vi "Segment Waveform Array.vi"(8 "error in (no error)":errorcluster caption="错误输入（无错误）", 10 "segment time":dbl=5.0 caption="分割时刻" format="%#_13g", 11 "original wavefrom array":waveform(dbl)[](array[waveform]) caption="原波形数组") -> (0 "error out":errorcluster caption="错误输出", 2 "waveform array part 0":waveform(dbl)[](array[waveform]) caption="波形数组前段", 3 "waveform array part 1":waveform(dbl)[](array[waveform]) caption="波形数组后段")   [LabVIEW 2015]
uses:
  <vilib>/Waveform/WDTOps.llb/WDT Waveform Duration DBL.vi
  <vilib>/Waveform/WDTOps.llb/WDT Get Waveform Subset DBL.vi
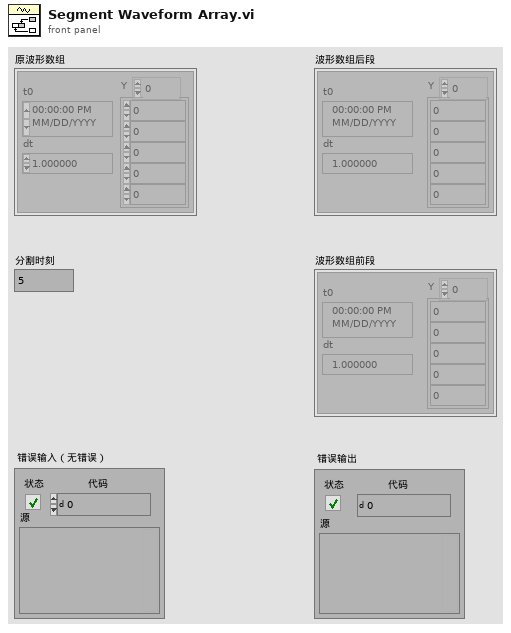
[diagram p1: front panel]
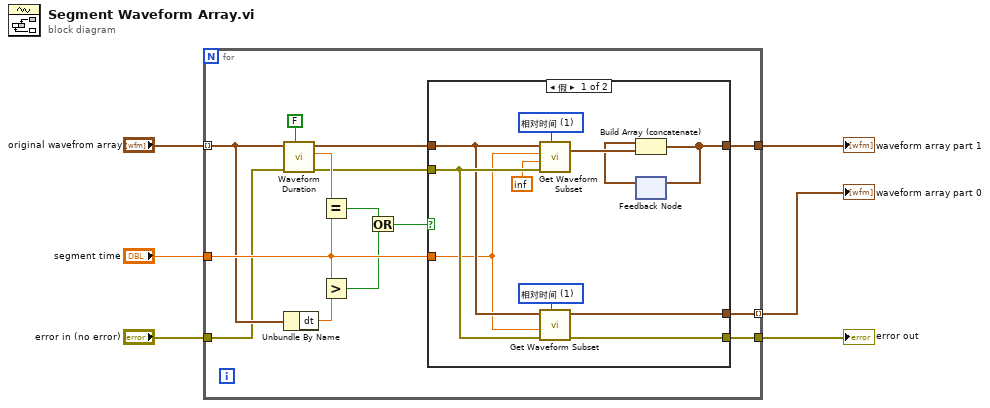
[diagram p0: block diagram]
diagram:
  n1 = for {
    tunnel: [w20] -> w4 mode=indexing
    tunnel: "original wavefrom array" -> [w10] mode=indexing
    tunnel: "error in (no error)" -> [w9]
    tunnel: [w19] -> w6
    tunnel: [w7] -> w1
    tunnel: "segment time" -> [w15]
    n2 = call-poly <vilib>:"Waveform Duration.vi"("open interval? (T)"=FALSE, "error in (no error)"=w9, "waveform in"=w10) -> ("error out"=w8:errorcluster, "duration"=w18:dbl, "waveform out"=w11:waveform(dbl))  [unwired: 6 in]
    n3 = Unbundle By Name(w10) -> ("dt"=w16:dbl)
    n4 = Equal?(x=w15, y=w18) -> (x = y?=w13:bool)
    n5 = Greater?(x=w16, y=w15) -> (0:w14:bool)
    n6 = Or(x=w13, y=w14) -> (x .or. y?=w12:bool)
    n7 = case shown="假" w12 {
      tunnel: [w31 w33] -> w20
      tunnel: [w21 _] -> w19
      tunnel: [w30 w32] -> w7
      tunnel: w11 -> [w26 w33]
      tunnel: w15 -> [w25 _]
      tunnel: w8 -> [w27 w32]
      frame False {
        w28 = u16 1 items=["采样", "相对时间"] ("start/duration format")
        w29 = u16 1 items=["采样", "相对时间"] ("start/duration format")
        n8 = call-poly <vilib>:"Get Waveform Subset.vi"("start/duration format"=w28, "error in (no error)"=w27, "duration"=inf, "start samples/time"=w25, "waveform in"=w26) -> ("waveform out"=w23:waveform(dbl))  [unwired: 1 in, 3 out]
        n9 = call-poly <vilib>:"Get Waveform Subset.vi"("start/duration format"=w29, "error in (no error)"=w27, "duration"=w25, "waveform in"=w26) -> ("error out"=w30:errorcluster, "waveform out"=w31:waveform(dbl))  [unwired: 2 in, 2 out]
        n10 = feedback #1() -> (w22:waveform(dbl)[])  [unwired: 1 in]
        n11 = Build Array (concatenate)(w22, w23) -> (w21:waveform(dbl)[])
        n12 = feedback-in #1(w21) -> ()
      }
      frame True {
      }
    }
  }
  "waveform array part 1" <- w6
  "waveform array part 0" <- w4
  "error out" <- w1
